vi "ReadTempVar.vi"(3 "error in":errorcluster, 4 "Name":string, 5 "storage refnum (file)":refnum<k20>) -> (0 "error out":errorcluster, 1 "Numeric Indicator":dbl, 2 "storage refnum (file) out":refnum<k20>)   [LabVIEW 2014]
uses:
  <vilib>/Platform/storage/lvStorage.llb/_queryPropPoly.vi
  <vilib>/Platform/storage/lvStorage.llb/_queryPropString.vi
  <vilib>/Platform/storage/lvStorage.llb/_queryGenericObjects.vi
  <vilib>/Platform/storage/lvStorage.llb/xStorage/xStorageSupp/ErrorOut.vi
  <vilib>/Platform/storage/lvStorage.llb/_loadAllDdt.vi
  <vilib>/Platform/storage/lvStorage.llb/xStorage/Read Data/Read Data.xnode
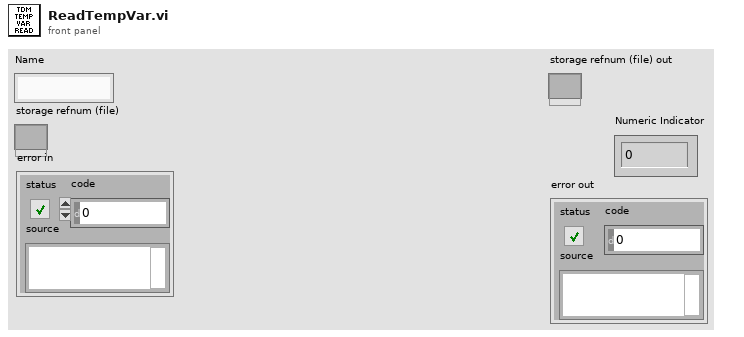
[diagram p1: front panel]
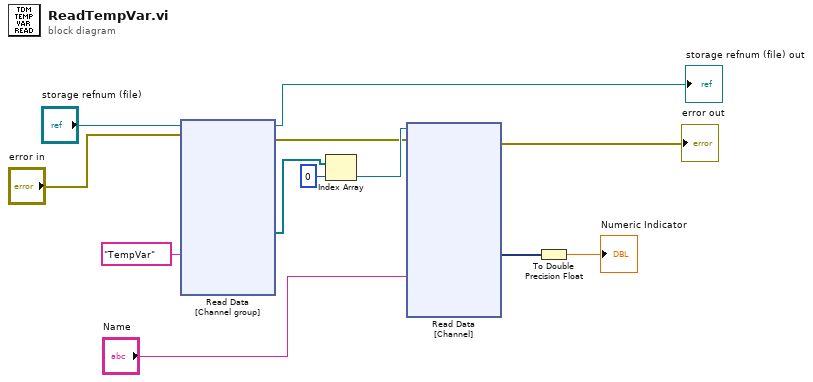
[diagram p0: block diagram]
diagram:
  n1 = xnode "Read Data\n[Channel group]"("Name"="TempVar", "storage refnum (file)"="storage refnum (file)", "error in"="error in") -> ("storage refnums (channel group)"=w10:refnum<k20>[], "storage refnum (file) out"=→"storage refnum (file) out":refnum<k20>, "error out"=w8:errorcluster)  [unwired: 1 in]
  n2 = Index Array(array=w10, index=0) -> (element=w9:refnum<k20>)
  n3 = xnode "Read Data\n[Channel]"("Name"="Name", "storage refnum (channel group)"=w9, "error in"=w8) -> ("Signal"=w6:dynamicdata, "error out"=→"error out":errorcluster)  [unwired: 3 in, 2 out]
  n4 = To Double Precision Float(number=w6) -> (double precision float=→"Numeric Indicator":dbl)
